vi "Example.vi"() -> ()   [LabVIEW 2014]
uses:
  ADIS16448.lvlib
  <vilib>/Rock Robotics/SystemInterfaces/DIO/FPGA_DIOChannel.ctl
panel:
  out "Waveform Chart":dbl(graph)
  out "Received Data":u8[](array[numeric]) format="%.0x"
  in  "stop 2":bool
  in  "stop":bool
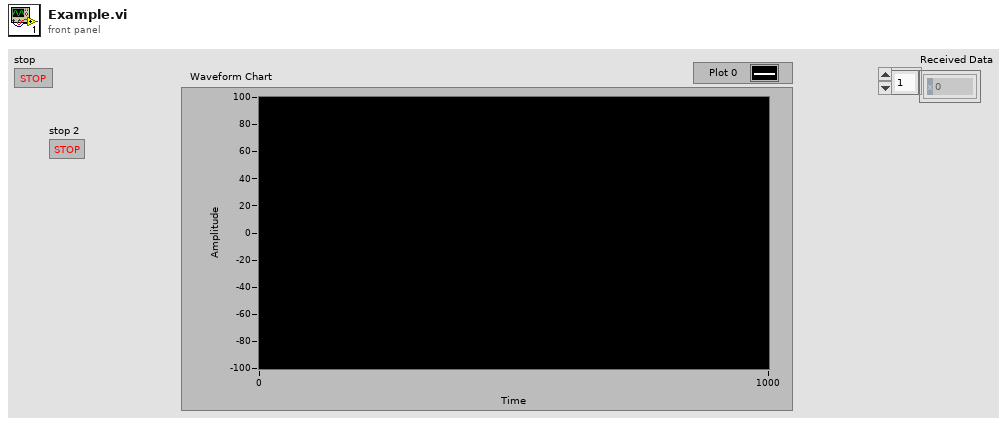
[diagram p1: front panel]
types:
  T1 = typedef "FPGA_DIOChannel.ctl" = enum8{"DIO 0", "DIO 1", "DIO 2", "DIO 3", "DIO 4", "DIO 5", "DIO 6", "DIO 7", "DIO 8", "DIO 9", "DIO MXP 0", "DIO MXP 1", "DIO MXP 2", "DIO MXP 3", "DIO MXP 4", "DIO MXP 5", "DIO MXP 6", "DIO MXP 7", "DIO MXP 8", "DIO MXP 9", "DIO MXP 10", "DIO MXP 11", "DIO MXP 12", "DIO MXP 13", "DIO MXP 14", "DIO MXP 15", "Invalid"}
  T2 = typedef "ADIS16448.lvlib/WPI_ADIS16448Ref.ctl" = cluster{"SPI Ref":T3, "DIO1 Digital Source Ref":T6, "DIO2 Digital Source Ref":T6, "DIO3 Digital Source Ref":T6, "DIO4 Digital Source Ref":T6, "Sample Mode":T10, "BurstMode":bool, "Registers to Read":T11[], "ReadingsDVR":T12, "GyroFactor":dbl, "InteruptRef":T13}
  T3 = typedef "WPI_SPIDevRef.ctl" = cluster{"DevStatus":errorcluster, "Handle":i32, "Controller":T4, "SPI Bus":T5}
  T4 = typedef "FPGA_TypedefDigitalModule.ctl" = enum16{"Controller 1"}
  T5 = typedef "spi_bus.ctl" = enum16{"SPI On-Board, CS0", "SPI On-Board, CS1", "SPI On-Board, CS2", "SPI On-Board, CS3", "SPI MXP", "Invalid"}
  T6 = typedef "FPGA_CounterEncoderSourceConvertionLVSourceType.ctl" = cluster{"DevStatus":errorcluster, "AnalogTriggerMode?":bool, "DigitalMode":cluster{"Controller":T4, "DIO Channel":T7}, "AnalogTriggerMode":cluster{"AnalogTriggerIndex":T8, "OutputType":T9}}
  T7 = typedef "FPGA_DIODigitalSourceChannel.ctl" = enum8{"DIO 0", "DIO 1", "DIO 2", "DIO 3", "DIO 4", "DIO 5", "DIO 6", "DIO 7", "DIO 8", "DIO 9", "DIO MXP 0", "DIO MXP 1", "DIO MXP 2", "DIO MXP 3", "DIO MXP 4", "DIO MXP 5", "DIO MXP 6", "DIO MXP 7", "DIO MXP 8", "DIO MXP 9", "DIO MXP 10", "DIO MXP 11", "DIO MXP 12", "DIO MXP 13", "DIO MXP 14", "DIO MXP 15", "Disabled"}
  T8 = typedef "FPGA_AnalogTriggerIndex.ctl" = enum8{"Trig 0", "Trig 1", "Trig 2", "Trig 3", "Trig 4", "Trig 5", "Trig 6", "Trig 7", "Invalid"}
  T9 = typedef "FPGA_AnalogTriggerOutType.ctl" = enum16{"InWindow", "TriggerState", "Rising", "Falling"}
  T10 = typedef "ADIS16448.lvlib/WPI_ADIS16448SampleMode.ctl" = enum16{"Interrupt", "Polled"}
  T11 = typedef "ADIS16448.lvlib/WPI_ADIS16448DataRegisters.ctl" = u16
  T12 = typedef "ADIS16448.lvlib/WPI_ADIS16448ReadingsDVR.ctl" = refnum<data-value>
  T13 = typedef "FPGA_InterruptRef.ctl" = cluster{"DevStatus":errorcluster, "Interrupt Index":T14}
  T14 = typedef "FPGA_InterruptIndex.ctl" = enum8{"0", "1", "2", "3", "4", "5", "6", "7", "Invalid"}
  T15 = typedef "WPI_DigitalInputDevRef.ctl" = cluster{"DevStatus":errorcluster, "DIO Channel":T1, "Controller":T4}
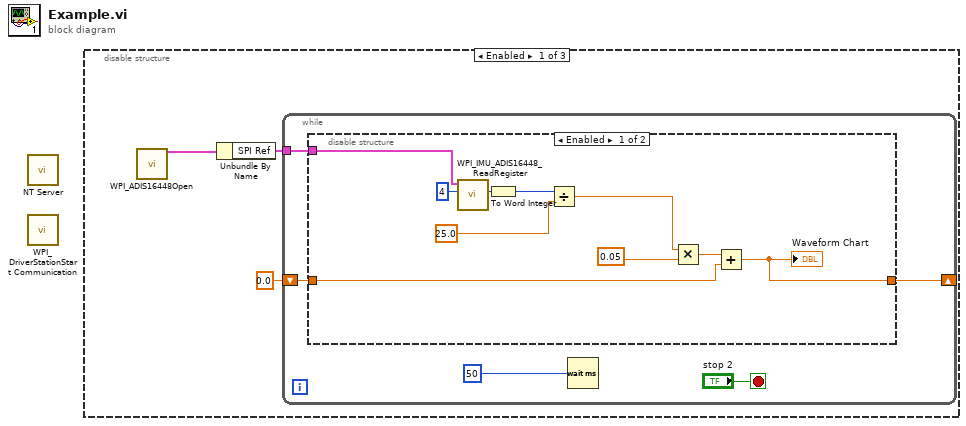
[diagram p0: block diagram]
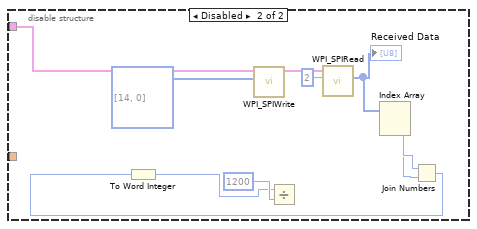
[diagram p2: hidden frame]
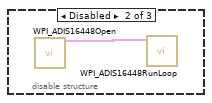
[diagram p3: hidden frame]
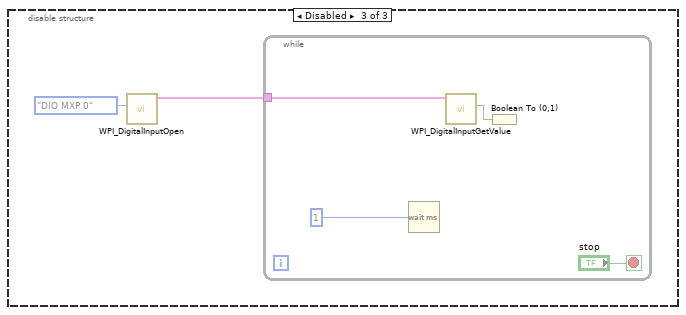
[diagram p4: hidden frame]
diagram:
  n1 = call <vilib>:"NT Server.vi"() -> ()  [unwired: 12 in]
  n2 = call <vilib>:"WPI_DriverStationStart Communication.vi"() -> ()  [unwired: 2 in, 10 out]
  n3 = disable-structure shown="Enabled" {
    frame Enabled {
      n4 = call "WPI_ADIS16448Open.vi"() -> ("ADIS16448DevRef"=w3:T2)  [unwired: 14 in, 1 out]
      n5 = Unbundle By Name(w3) -> ("SPI Ref"=w2:T3)
      n6 = while {
        tunnel: w2 -> [w8]
        shift-right: [w4] -> _
        shift-left: 0.0 -> [w5]
        stop <- "stop 2" stop-if-true
        n7 = disable-structure shown="Enabled" {
          disable-tunnel: w8 -> [w17 w29]
          disable-tunnel: w5 -> [w9 _]
          disable-tunnel: [w10 _] -> w4
          frame Enabled {
            n8 = call "WPI_IMU_ADIS16448_ReadRegister.vi"("Register"=u8 4, "SPIDevRef in"=w17) -> ("Register Value"=w16:u16)  [unwired: 7 in, 2 out]
            n9 = To Word Integer(number=w16) -> (16bit integer=w14:i16)
            n10 = Divide(x=w14, y=25.0) -> (x/y=w12:dbl)
            n11 = Multiply(x=w12, y=0.05) -> (x*y=w11:dbl)
            n12 = Add(x=w11, y=w9) -> (x+y=w10:dbl)
            "Waveform Chart" <- w10
          }
          frame Disabled {
            n13 = call <vilib>:"WPI_SPIWrite.vi"("Data To Send"=u8[] [14, 0], "SPIDevRef"=w29) -> ("SPIDevRef"=w27:T3)  [unwired: 7 in, 2 out]
            n14 = call <vilib>:"WPI_SPIRead.vi"("Num to Read"=2, "SPIDevRef"=w27) -> ("Received Data"=w25:u8[])  [unwired: 7 in, 2 out]
            "Received Data" <- w25
            n15 = Index Array(array=w25) -> (element #1=w24:u8, element #2=w23:u8)  [unwired: 2 in]
            n16 = Join Numbers(hi=w24, lo=w23) -> ((hi.lo)=w20:u16)
            n17 = To Word Integer(number=w20) -> (16bit integer=w19:i16)
            n18 = Divide(x=w19, y=i16 1200) -> (x/y=w21:dbl)
          }
        }
        n19 = Wait (ms)(milliseconds to wait=u32 50) -> ()  [unwired: 1 out]
      }
    }
    frame Disabled {
      n20 = call "WPI_ADIS16448Open.vi"() -> ("ADIS16448DevRef"=w30:T2)  [unwired: 14 in, 1 out]
      n21 = call "WPI_ADIS16448RunLoop.vi"("ADIS16448DevRef in"=w30) -> ()  [unwired: 9 in, 2 out]
    }
    frame Disabled {
      n22 = call <vilib>:"WPI_DigitalInputOpen.vi"("DIO Channel"=FPGA_DIOChannel."DIO MXP 0") -> ("DigitalInputDevRef"=w32:T15)  [unwired: 9 in, 1 out]
      n23 = while {
        tunnel: w32 -> [w37]
        stop <- "stop" stop-if-true
        n24 = Wait (ms)(milliseconds to wait=u32 1) -> ()  [unwired: 1 out]
        n25 = call <vilib>:"WPI_DigitalInputGetValue.vi"("DigitalInputDevRef"=w37) -> ("Value"=w35:bool)  [unwired: 8 in, 2 out]
        n26 = Boolean To (0,1)(Boolean=w35) -> (0, 1=w34:i16)
      }
    }
  }
